vi "MBT_SaveToLogFile.vi"(8 "error in":errorcluster, 10 "path":path, 11 "MulticolumnListbox in":refnum<vi>) -> (0 "error out":errorcluster)   [LabVIEW 2012, in "MBT_ModbusTester.lvlib"]
uses:
  MBT_ModbusTester.lvlib
  <vilib>/Utility/file.llb/Write To Spreadsheet File (string).vi
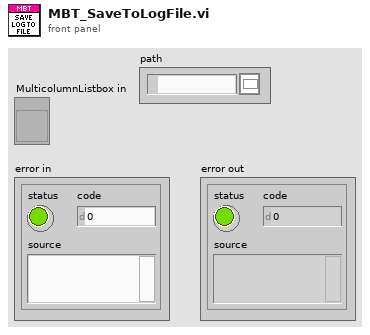
[diagram p1: front panel]
types:
  T1 = enum16{"open", "replace", "create", "open or create", "replace or create", "replace or create with confirmation"}
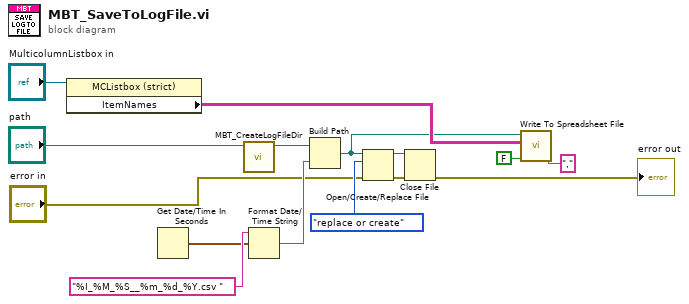
[diagram p0: block diagram]
diagram:
  n1 = property on="Property Node" class="MCListbox (strict)"(reference="MulticolumnListbox in") -> ("ItemNames"=w13:string[][])  [unwired: 1 in, 2 out]
  n2 = Get Date/Time In Seconds() -> (seconds since 1Jan1904=w5:timestamp)
  n3 = call "MBT_CreateLogFileDir.vi"("path"="path") -> ("appended path"=w2:path)  [unwired: 10 in]
  n4 = Format Date/Time String(time format string (%c)="%I_%M_%S__%m_%d_%Y.csv ", seconds (now)=w5) -> (date/time string=w7:string)  [unwired: 1 in]
  n5 = Build Path(base path=w2, name or relative path=w7) -> (appended path=w12:path)
  n6 = Open/Create/Replace File(file path (use dialog)=w12, error in="error in", operation (0:open)=T1."replace or create") -> (refnum out=w10:refnum<file>, error out=w11:errorcluster)  [unwired: 3 in, 1 out]
  n7 = Close File(refnum=w10, error in=w11) -> (error out=→"error out":errorcluster)  [unwired: 1 out]
  n8 = call-poly <vilib>:"Write To Spreadsheet File.vi"("delimiter (\\t)"="," ("delimiter (\\t)"), "append to file? (new file:F)"=FALSE, "2D data"=w13, "file path (dialog if empty)"=w12) -> ()  [unwired: 4 in, 1 out]
